vi "oa_Create CIC Compensation Filter.vi"(4 "CIC stages":i32[](array[numeric])=[4, 6, 8], 6 "alias protect in final transition":bool, 9 "stop band attenuation":u16(ring)=2 items=["72 dB", "96 dB", "120 dB"], 11 "decimation factor":i32) -> (1 "stage":i32, 3 "compensation filter settings":T1={"coefficients"=[], "factor"=1} {"coefficients" format="%.2f"})   [LabVIEW 2017, in "SoundVib_Resampling.lvlib"]
uses:
  <vilib>/addons/Sound and Vibration/Order Analysis/Resample Order Tracking/SoundVib_Resampling.lvlib
  <vilib>/addons/_NISVFA/_Shared subVIs/Controls/OAT Decimation Filter.ctl
  <vilib>/Analysis/1siggen.llb/Ramp Pattern by Samples.vi
  <vilib>/Analysis/2dsp.llb/Real FFT.vi
  <vilib>/Analysis/NI_AALBase.lvlib
  <vilib>/Analysis/NI_AALPro.lvlib
panel:
  in  "Case Constant\n(See Context Help)":bool
  in  "linear/log":bool
  out "frequency response":cluster{"Element Data":dbl, dbl, dbl[]}(graph)={"Element Data"=0.0, 1.52587890625e-05, []}
  out "pass band error":dbl[](graph)
  in  "WEIGHT":dbl=10.0 format="%.2f"
  in  "#of compensation points":i32=30
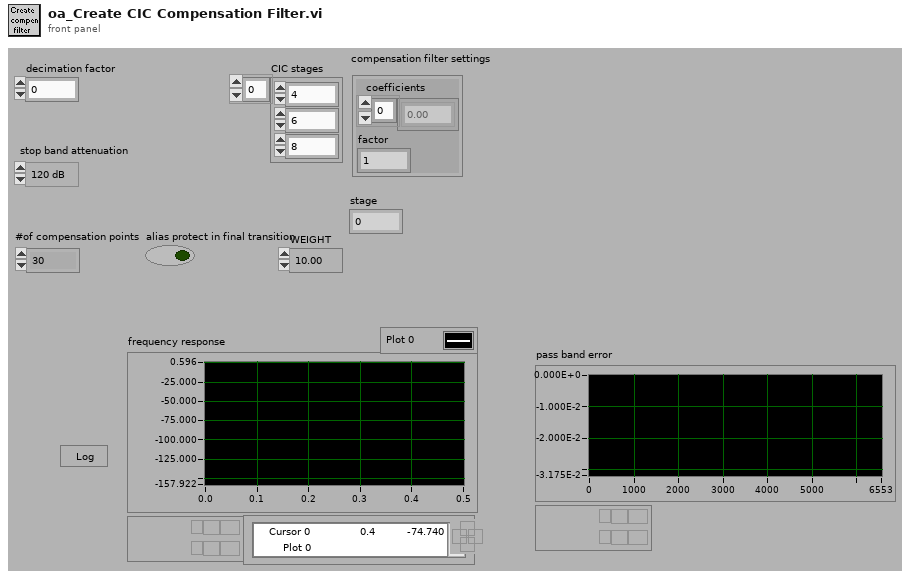
[diagram p1: front panel]
types:
  T1 = typedef "OAT Decimation Filter.ctl" = cluster{"coefficients":dbl[], "factor":i32}
  T2 = cluster{"Element Data":dbl, "Element Data":dbl, "Element Data":dbl, "WEIGHT":dbl}[]
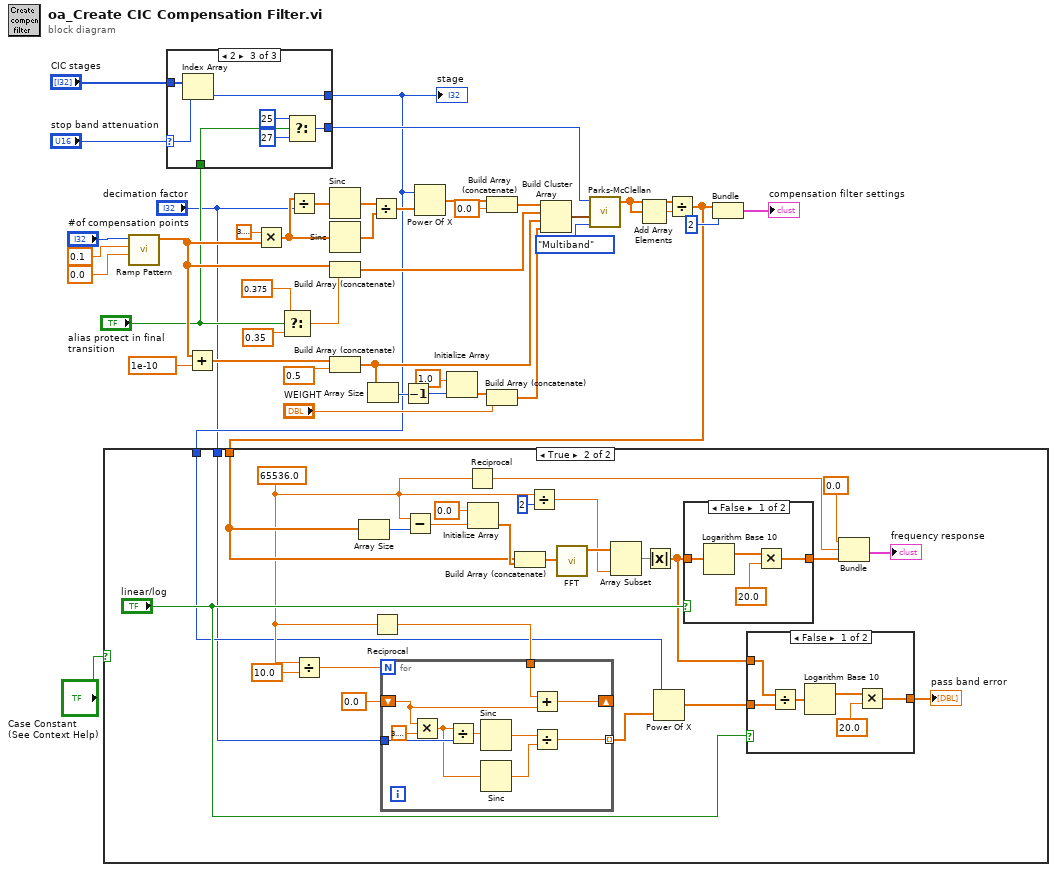
[diagram p0: block diagram]
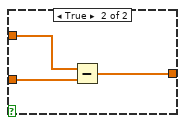
[diagram p3: hidden frame]
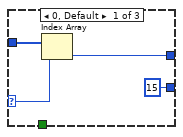
[diagram p5: hidden frame]
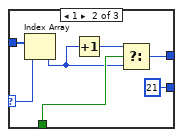
[diagram p6: hidden frame]
diagram:
  n1 = call-poly <vilib>:"Ramp Pattern.vi"("start"=0.0, "end"=0.1, "samples"="#of compensation points") -> ("Ramp Pattern"=w23:dbl[])  [unwired: 7 in, 1 out]
  n2 = case shown="2" "stop band attenuation" {
    selector: "stop band attenuation" -> [w43 w48 w54]
    tunnel: [w42 w50 w53] -> w7
    tunnel: [15 21 w57] -> w12
    tunnel: "alias protect in final transition" -> [_ w51 w59]
    tunnel: "CIC stages" -> [w44 w49 w55]
    frame 0, Default {
      n3 = Index Array(array=w44, index=w43) -> (element=w42:i32)
    }
    frame 1 {
      n4 = Index Array(array=w49, index=w48) -> (element=w46:i32)
      n5 = Increment(x=w46) -> (x+1=w47:i32)
      n6 = Select(t=w47, s=w51, f=w46) -> (s? t:f=w50:i32)
    }
    frame 2 {
      n7 = Index Array(array=w55, index=w54) -> (element=w53:i32)
      n8 = Select(t=25, s=w59, f=27) -> (s? t:f=w57:i32)
    }
  }
  "stage" <- w7
  n9 = Add(x=w23, y=1e-10 ("Element Data")) -> (x+y=w32:dbl[])
  n10 = Multiply(x=3.141592653589793, y=w23) -> (x*y=w24:dbl[])
  n11 = Select(t=0.375 ("Element Data"), s="alias protect in final transition", f=0.35 ("Element Data")) -> (s? t:f=w9:dbl)
  n12 = Divide(x=w24, y="decimation factor") -> (x/y=w25:dbl[])
  n13 = Sinc(1:w25) -> (0:w22:dbl[])
  n14 = Sinc(1:w24) -> (0:w15:dbl[])
  n15 = Build Array (concatenate)(w23, w9) -> (w33:dbl[])
  n16 = Build Array (concatenate)(w32, 0.5 ("Element Data")) -> (w29:dbl[])
  n17 = Array Size(array=w29) -> (size(s)=w38:i32)
  n18 = Divide(x=w22, y=w15) -> (x/y=w21:dbl[])
  n19 = Decrement(x=w38) -> (x-1=w20:i32)
  n20 = Power Of X(1:w21, 2:w7) -> (0:w16:dbl[])
  n21 = Initialize Array(1.0 ("Element Data"), w20) -> (w36:dbl[])
  n22 = Build Array (concatenate)(w16, 0.0 ("Element Data")) -> (w17:dbl[])
  n23 = Build Array (concatenate)(w36, "WEIGHT") -> (w19:dbl[])
  n24 = Build Cluster Array(w17, w33, w29, w19) -> (w34:T2)
  n25 = call <vilib>:"Parks-McClellan.vi"("filter type"=enum32{"Multiband", "Differentiator", "Hilbert"}."Multiband", "Band Parameters"=w34, "# of taps"=w12) -> ("h"=w3:dbl[])  [unwired: 1 in, 2 out]
  n26 = Add Array Elements(numeric array=w3) -> (sum=w4:dbl)
  n27 = Divide(x=w3, y=w4) -> (x/y=w2:dbl[])
  n28 = case shown="True" "Case Constant\n(See Context Help)" {
    tunnel: w2 -> [_ w68]
    tunnel: w7 -> [_ w61]
    tunnel: "decimation factor" -> [_ w60]
    frame False {
    }
    frame True {
      w66 = 65536.0 ("Element Data")
      n29 = Divide(x=w66, y=10.0) -> (x/y=w67:dbl)
      n30 = Array Size(array=w68) -> (size(s)=w82:i32)
      n31 = Reciprocal(x=w66) -> (1/x=w62:dbl)
      n32 = for {
        N: w67 -> [_]
        shift-right: [w87] -> _
        shift-left: 0.0 -> [w88]
        tunnel: w60 -> [w94]
        tunnel: [w89] -> w63 mode=indexing
        tunnel: w62 -> [w86]
        n33 = Multiply(x=w88, y=3.141592653589793) -> (x*y=w92:dbl)
        n34 = Divide(x=w92, y=w94) -> (x/y=w93:dbl)
        n35 = Sinc(1:w93) -> (0:w91:dbl)
        n36 = Sinc(1:w92) -> (0:w90:dbl)
        n37 = Add(x=w86, y=w88) -> (x+y=w87:dbl)
        n38 = Divide(x=w91, y=w90) -> (x/y=w89:dbl)
      }
      n39 = Subtract(x=w66, y=w82) -> (x-y=w77:dbl)
      n40 = Reciprocal(x=w66) -> (1/x=w73:dbl)
      n41 = Initialize Array(0.0 ("Element Data"), w77) -> (w84:dbl[])
      n42 = Build Array (concatenate)(w68, w84) -> (w76:dbl[])
      n43 = Divide(x=w66, y=2) -> (x/y=w80:dbl)
      n44 = call-poly <vilib>:"FFT.vi"("X"=w76) -> ("FFT {X}"=w83:cdb[])  [unwired: 9 in, 1 out]
      n45 = Array Subset(array=w83, length=w80) -> (w79:cdb[])  [unwired: 1 in]
      n46 = Absolute Value(x=w79) -> (abs(x)=w69:dbl[])
      n47 = Power Of X(1:w63, 2:w61) -> (0:w70:dbl[])
      n48 = case shown="False" "linear/log" {
        tunnel: w69 -> [w108 w109]
        tunnel: [w107 w109] -> w74
        frame False {
          n49 = Logarithm Base 10(1:w108) -> (0:w106:dbl[])
          n50 = Multiply(x=w106, y=20.0 ("Element Data")) -> (x*y=w107:dbl[])
        }
        frame True {
        }
      }
      n51 = case shown="False" "linear/log" {
        tunnel: [w101 w102] -> w71
        tunnel: w69 -> [w97 w104]
        tunnel: w70 -> [w96 w103]
        frame False {
          n52 = Divide(x=w97, y=w96) -> (x/y=w98:dbl[])
          n53 = Logarithm Base 10(1:w98) -> (0:w100:dbl[])
          n54 = Multiply(x=w100, y=20.0 ("Element Data")) -> (x*y=w101:dbl[])
        }
        frame True {
          n55 = Subtract(x=w104, y=w103) -> (x-y=w102:dbl[])
        }
      }
      "pass band error" <- w71
      n56 = Bundle("Element Data"=0.0, w73, w74) -> (→"frequency response":cluster{"Element Data":dbl, dbl, dbl[]})  [unwired: 1 in]
    }
  }
  n57 = Bundle(w2, 2) -> (→"compensation filter settings":cluster{dbl[], i32})  [unwired: 1 in]
